vi "Process.vi"(8 "error in":errorcluster, 11 "SMO.A":refnum<class "SMO.Configurable.lvclass">) -> (0 "error out":errorcluster, 3 "SMO.A out":refnum<class "SMO.Configurable.lvclass">)   [LabVIEW 2013, in "SMO.Configurable.lvclass"]
doc: "---------------------------------------------------------------\nJKI State Machine Objects™\nhttp://jki.net/state-machine-objects/\nCopyright (C) 2005-2015, JKI <info@jki.net>\nALL RIGHTS RESERVED"
uses:
  SMO.Configurable.lvclass
  src/SMO/Typedefs/Parent Call--Enum.ctl
  src/SMO/SMO.lvclass
panel:
  # "For instructions on how to use the JKI State Machine Objects, examples and video tutorials, visit:\nhttp://jki.net/state-machine-objects/\n\nJKI State Machine Objects™\nhttp://jki.net/state-machine-objects/\nCopyright (C) 2005-2015, JKI <info@jki.net>\nALL RIGHTS RESERVED"
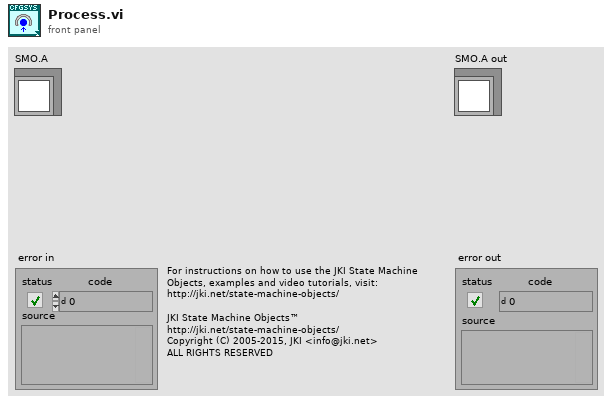
[diagram p1: front panel]
types:
  T1 = typedef "SMO.lvclass/Parent Call--Enum.ctl" = enum16{"Allows parent to run", "Does not request parent to run"}
  T2 = enum32{"invalid app kind", "Development System", "Run Time System", "Student Edition", "Embedded LabVIEW", "Evaluation", "Custom"}
  T3 = enum32{"Invalid", "Standard", "Closed", "Hidden", "Minimized", "Maximized"}
  T4 = cluster{"Core":cluster{"Current VI Reference":refnum<vi>, "Close Panel on Exit?":bool, "error":errorcluster}, "Self Ref":refnum<class "SMO.Configurable.lvclass">, "timeout":i32, "start time":timestamp}
  T5 = cluster{"Current VI Reference":refnum<vi>, "Close Panel on Exit?":bool, "error":errorcluster}
  T6 = typedef "SMO.Configurable.lvclass/Config--cluster.ctl" = cluster{"timeout":i32, "run":bool}
  T7 = typedef "SMO.lvclass/Protected Events.ctl" = cluster{"StopProcesses":refnum<user-event>, "AbortProcesses":refnum<user-event>, "Config Changed":refnum<user-event>, "Dependency":refnum<user-event>}
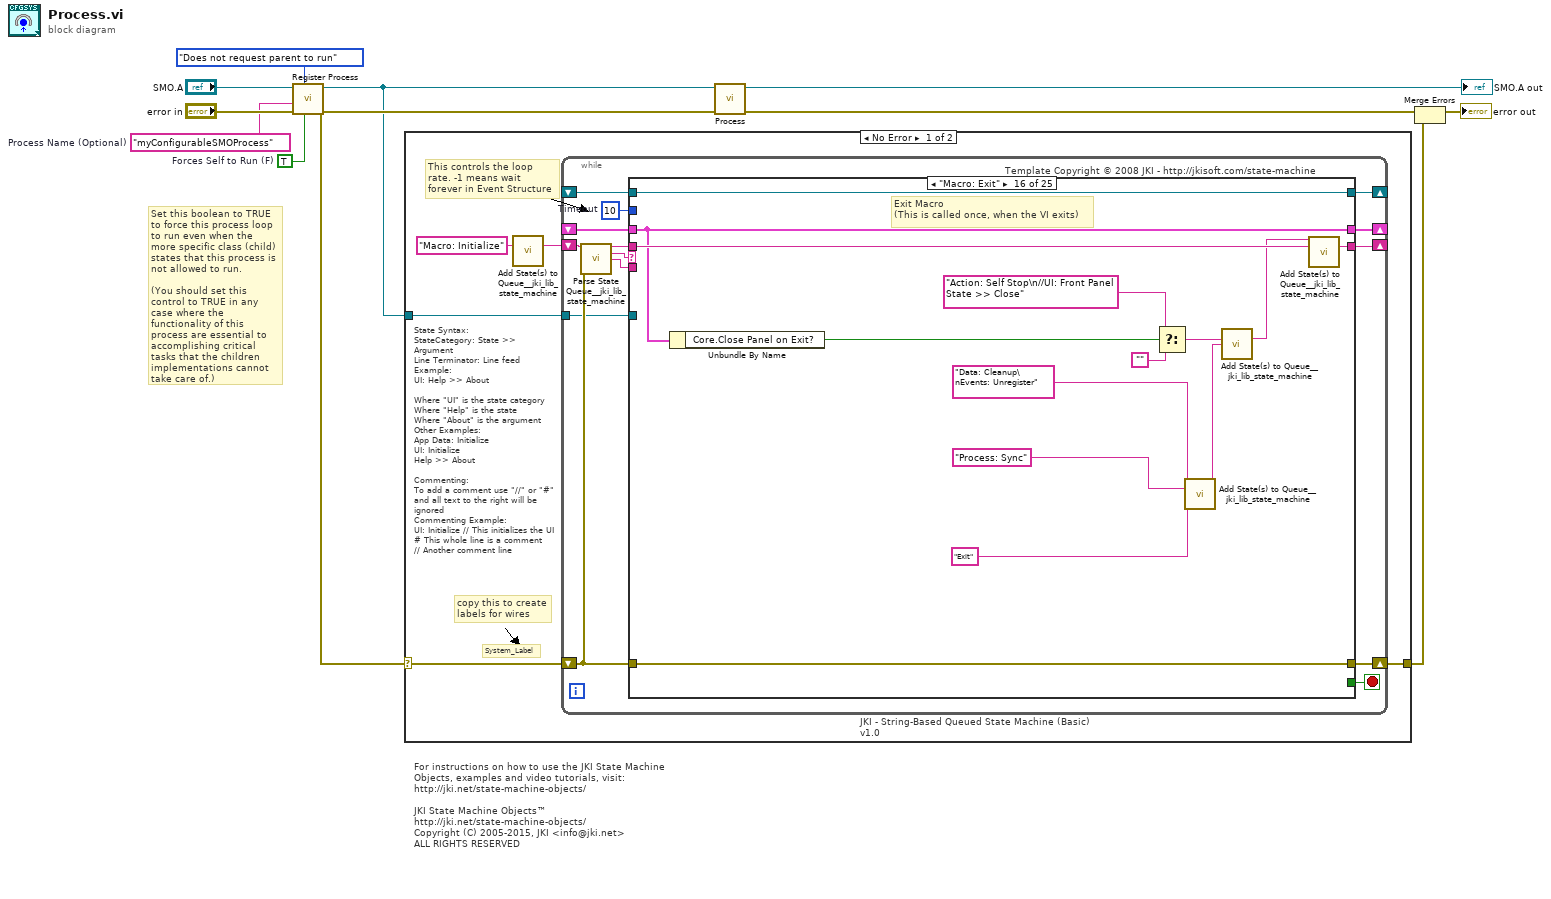
[diagram p0: block diagram]
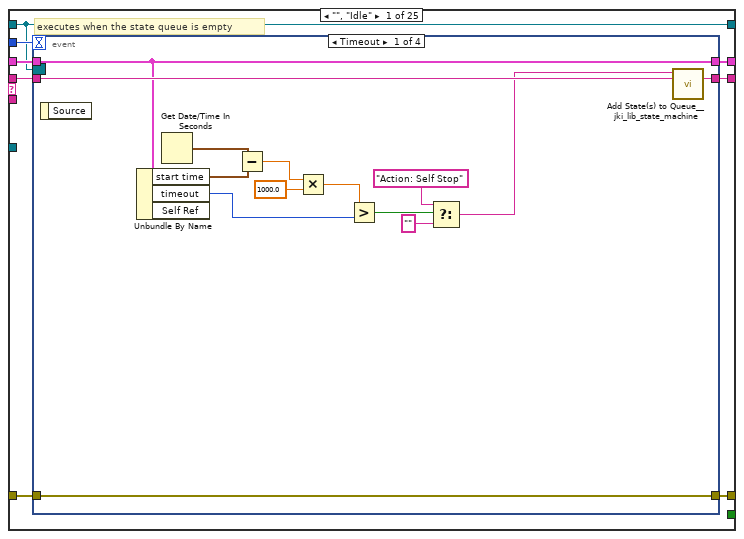
[diagram p2: hidden frame]
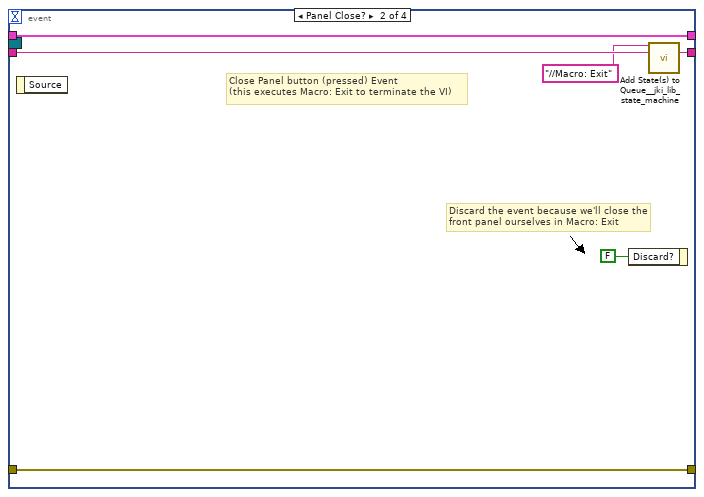
[diagram p3: hidden frame]
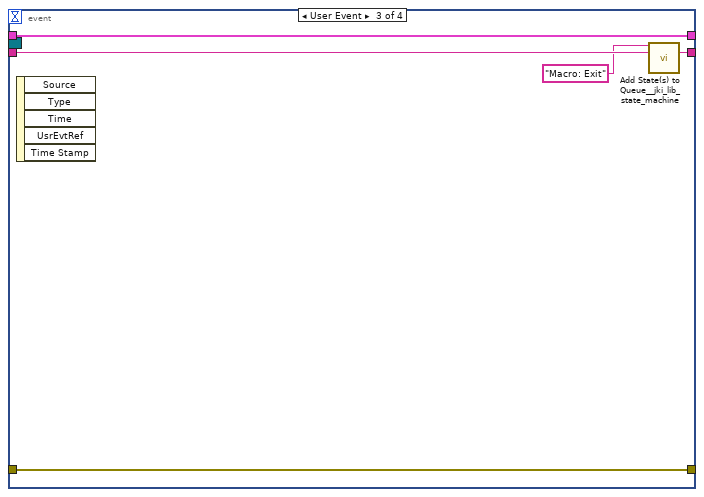
[diagram p4: hidden frame]
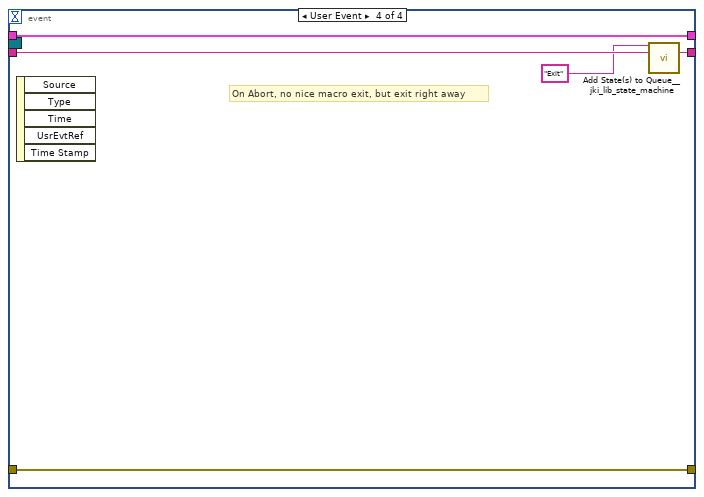
[diagram p5: hidden frame]
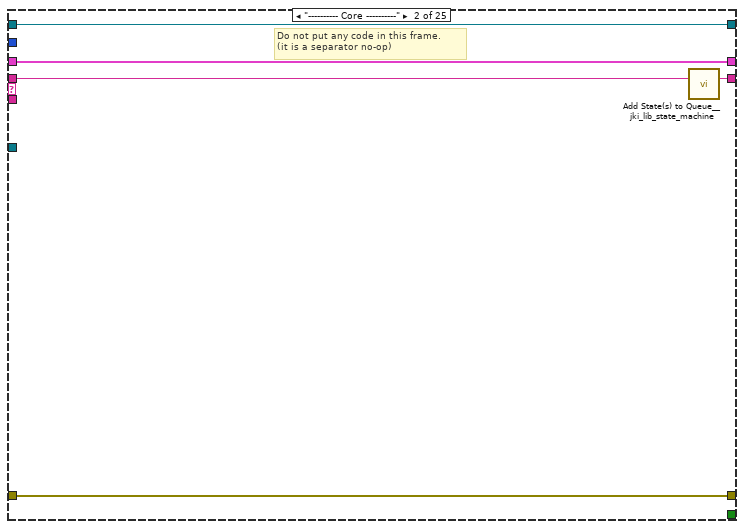
[diagram p6: hidden frame]
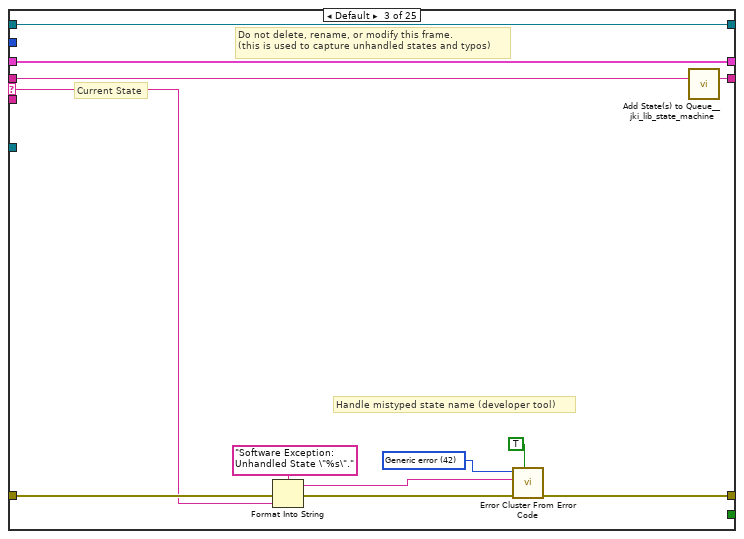
[diagram p7: hidden frame]
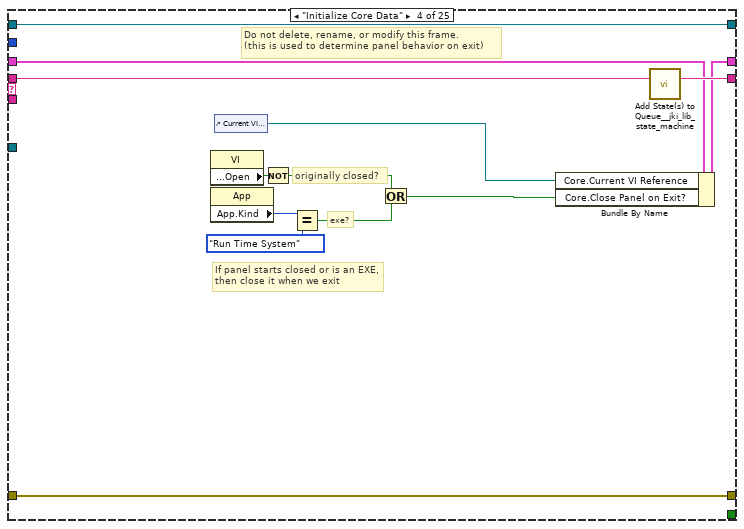
[diagram p8: hidden frame]
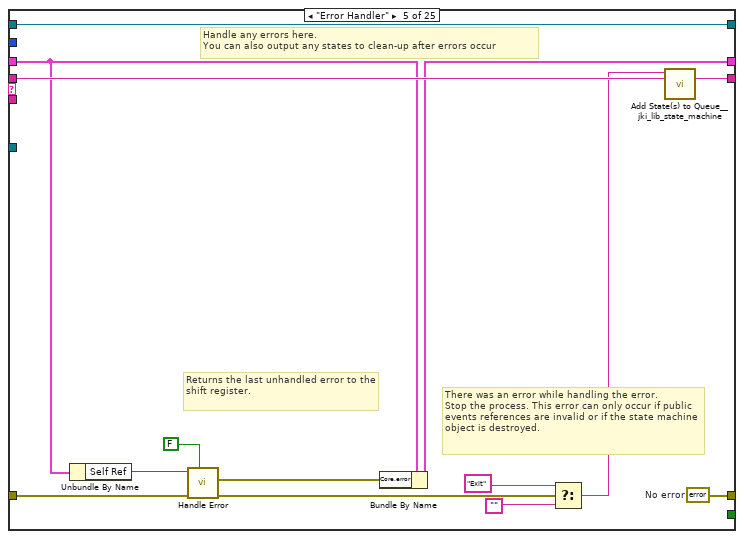
[diagram p9: hidden frame]
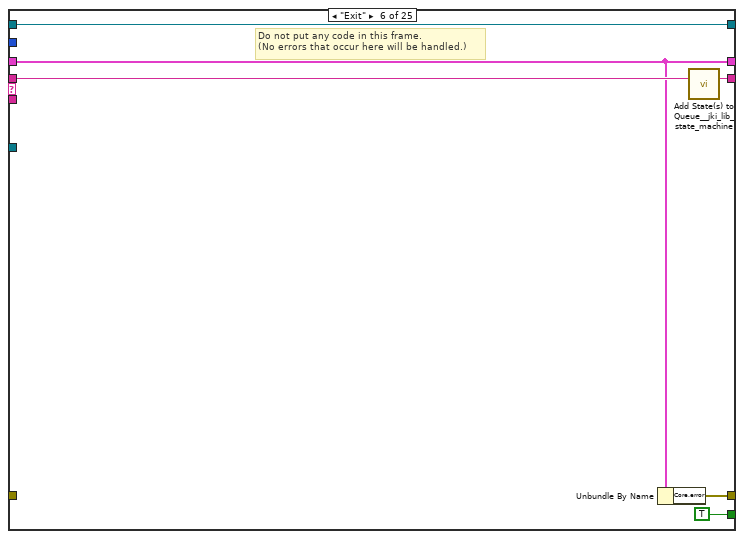
[diagram p10: hidden frame]
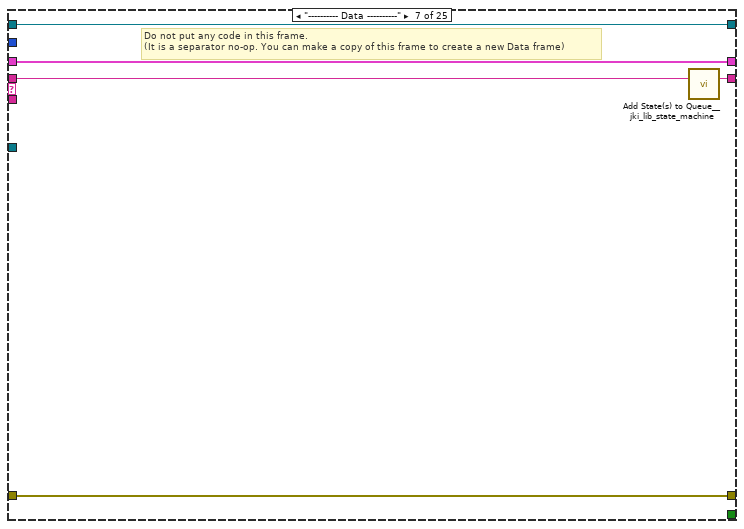
[diagram p11: hidden frame]
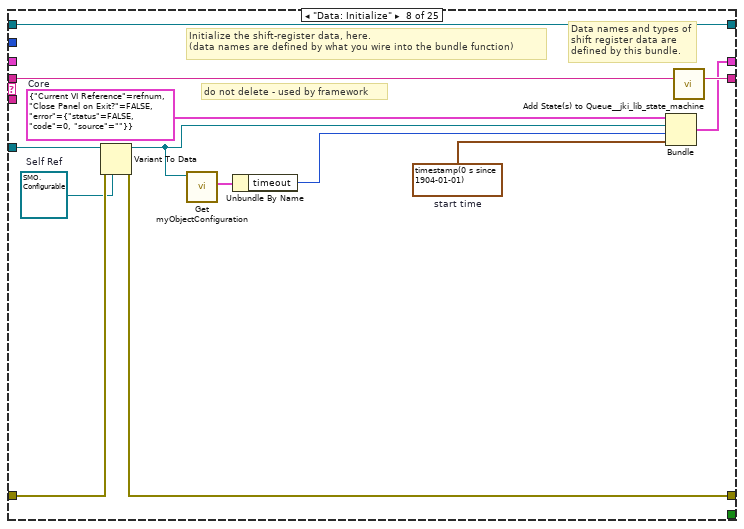
[diagram p12: hidden frame]
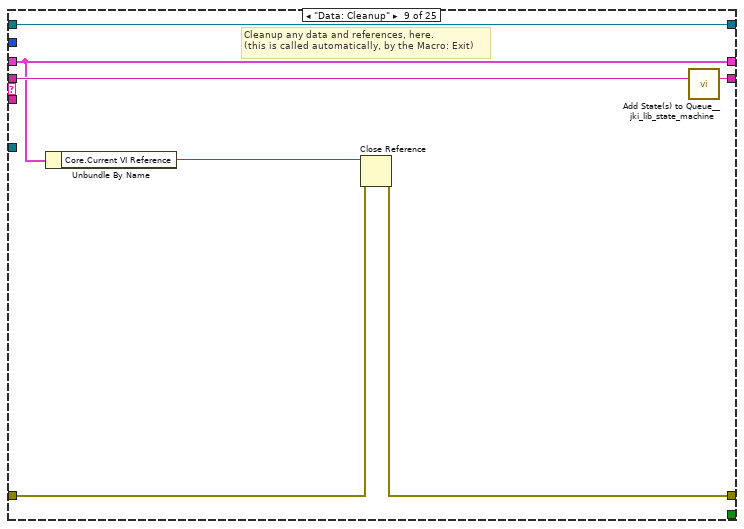
[diagram p13: hidden frame]
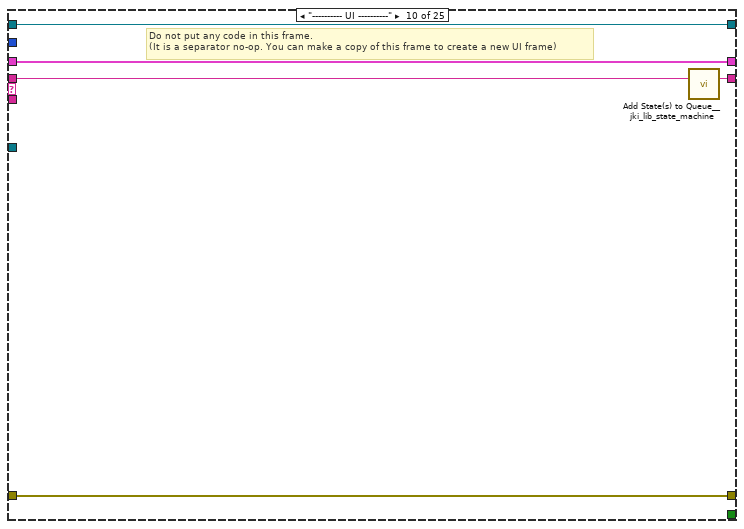
[diagram p14: hidden frame]
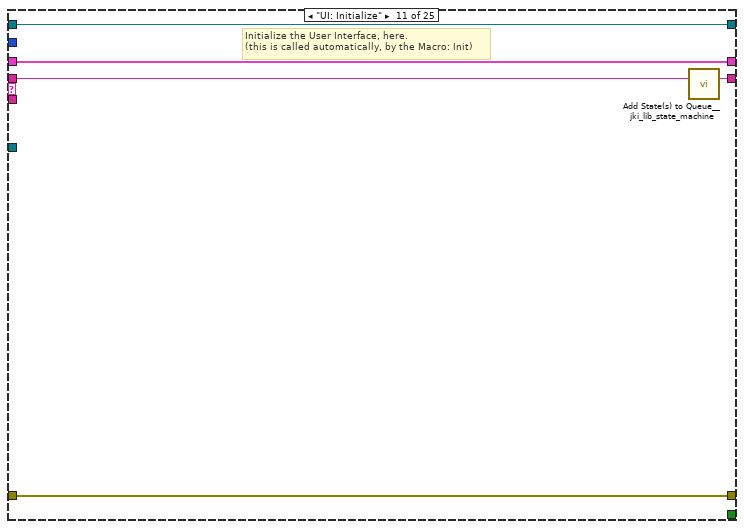
[diagram p15: hidden frame]
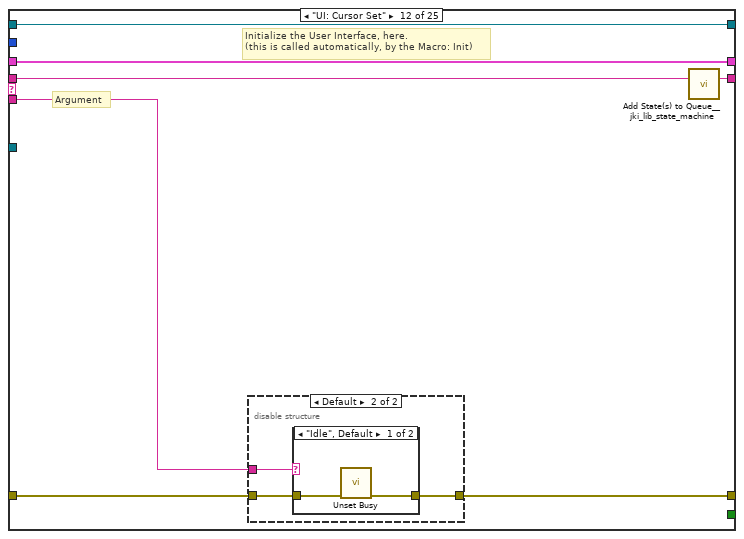
[diagram p16: hidden frame]
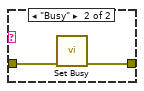
[diagram p18: hidden frame]
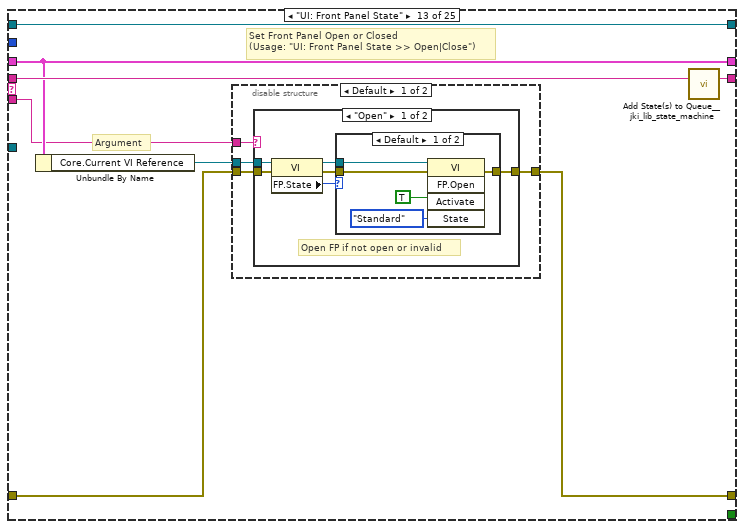
[diagram p19: hidden frame]
diagram:
  w1 = TRUE  # Forces Self to Run (F)
  w2 = "myConfigurableSMOProcess"  # Process Name (Optional)
  # "Set this boolean to TRUE to force this process loop to run even when the more specific class (child) states that this process is not allowed to run.\n\n(You should set this control to TRUE in any case where the functionality of this process are essential to accomplishing critical tasks that the children implementations cannot take care of.)"
  # "For instructions on how to use the JKI State Machine Objects, examples and video tutorials, visit:\nhttp://jki.net/state-machine-objects/\n\nJKI State Machine Objects™\nhttp://jki.net/state-machine-objects/\nCopyright (C) 2005-2015, JKI <info@jki.net>\nALL RIGHTS RESERVED"
  n1 = call "Register Process.vi"("Forces Self to Run (F)"=w1, "Parent Call"=Parent_Call--Enum."Does not request parent to run", "error in (no error)"="error in", "Process Name (optional)"=w2, "SMO"="SMO.A") -> ("error out"=w8:errorcluster, "SMO out"=w7:refnum<class "SMO.Configurable.lvclass">)  [unwired: 5 in]
  n2 = case shown="No Error" w8 {
    selector: w8 -> [w13 w301]
    tunnel: w7 -> [w14 _]
    tunnel: [w12 w301] -> w4
    frame No Error {
      # "State Syntax:\nStateCategory: State >> Argument\nLine Terminator: Line feed\nExample:\nUI: Help >> About\n\nWhere \"UI\" is the state category\nWhere \"Help\" is the state\nWhere \"About\" is the argument\nOther Examples:\nApp Data: Initialize\nUI: Initialize\nHelp >> About\n\nCommenting:\nTo add a comment use \"//\" or \"#\" and all text to the right will be ignored\nCommenting Example:\nUI: Initialize // This initializes the UI\n# This whole line is a comment\n// Another comment line"
      # "copy this to create labels for wires"
      # "This controls the loop rate. -1 means wait forever in Event Structure"
      # "System_Label"
      n3 = call <vilib>:"Add State(s) to Queue__jki_lib_state_machine.vi"("State(s) in (\"\")"="Macro: Initialize") -> ("States Out"=w16:string)  [unwired: 14 in]
      n4 = while "JKI - String-Based Queued State Machine (Basic) v1.0" {
        shift-right: [w23] -> _
        shift-left: _ -> [w22]
        shift-right: [w26] -> w12
        shift-left: w13 -> [w20]
        shift-right: [w25] -> _
        shift-left: w16 -> [w27]
        tunnel: w14 -> [w19]
        shift-right: [w18] -> _
        shift-left: _ -> [w17]
        stop <- w24 stop-if-true
        w21 = 10  # Timeout
        # "Template Copyright © 2008 JKI - http://jkisoft.com/state-machine"
        n5 = call <vilib>:"Parse State Queue__jki_lib_state_machine.vi"("State Queue"=w27, "Error In (no error)"=w20) -> ("Remaining States"=w29:string, "Current State"=w30:string, "Arguments"=w28:string)  [unwired: 11 in]
        n6 = case shown="\"Macro: Exit\"" w30 {
          selector: w30 -> [_ _ w75 _ _ _ _ _ _ _ _ _ _ _ _ _ _ _ _ _ _ _ _ _ _]
          tunnel: w29 -> [w38 w73 w79 w98 w112 w118 w123 w136 w143 w148 w153 w160 w176 w208 w217 w231 w236 w247 w252 w262 w268 w273 w280 w292 w300]
          tunnel: w28 -> [_ _ _ _ _ _ _ _ _ _ _ w154 w169 _ _ _ _ _ _ _ _ _ _ _ _]
          tunnel: w22 -> [w36 w70 w77 w89 w103 w114 w120 _ w138 w145 w151 w158 w174 w205 w213 w222 w233 w244 w249 w260 w266 w271 w275 w289 w297]
          tunnel: [w35 w71 w81 w95 w100 w113 w121 w132 w139 w146 w150 w155 w170 w206 w215 w229 w234 w238 w250 w254 w264 w269 w277 w281 w294] -> w26
          tunnel: w20 -> [w34 w71 w80 w95 w104 _ w121 w133 w140 w146 w150 w156 w171 w206 w215 w229 w234 w239 w250 w255 w264 w269 w277 w282 w295]
          tunnel: [w37 w72 w78 w97 w111 w117 w122 w135 w142 w147 w152 w159 w175 w207 w216 w230 w235 w246 w251 w261 w267 w272 w279 w291 w299] -> w25
          tunnel: [_ _ _ _ _ TRUE _ _ _ _ _ _ _ _ _ _ _ _ _ _ _ _ _ _ _] -> w24
          tunnel: [w33 w70 w77 w96 w102 w114 w120 w134 w138 w145 w151 w158 w174 w205 w213 w222 w233 w244 w249 w260 w266 w271 w274 w289 w297] -> w23
          tunnel: w21 -> [w32 _ _ _ _ _ _ _ _ _ _ _ _ _ _ _ _ _ _ _ _ _ _ _ _]
          tunnel: w19 -> [_ _ _ _ _ _ _ w130 _ _ _ _ _ _ _ _ _ _ _ _ _ _ _ _ _]
          tunnel: [w31 w69 w74 w86 w110 w115 w119 w129 w137 w144 w149 w157 w173 w204 w214 w223 w232 w245 w248 w258 w265 w270 w278 w290 w298] -> w18
          tunnel: w17 -> [w31 w69 w74 w86 w110 w115 w119 w129 w137 w144 w149 w157 w173 w204 w214 w223 w232 w245 w248 _ w265 w270 w278 w290 w298]
          frame "", "Idle" {
            # "executes when the state queue is empty"
            n7 = event shown="[0] Timeout" {
              selector: w31 -> [_ _ _ _]
              dyn-events: _ -> [_ _ _ _]
              timeout: w32 -> [_ _ _ _]
              tunnel: w38 -> [w52 w58 w63 w68]
              tunnel: [w51 w57 w62 w67] -> w37
              tunnel: w36 -> [w49 w55 w60 w65]
              tunnel: [w50 w56 w61 w66] -> w35
              tunnel: w34 -> [w50 w56 w61 w66]
              tunnel: [w49 w55 w60 w65] -> w33
              event Timeout {
                n8 = event-data() -> ()  [unwired: 1 in, 1 out]
                n9 = Unbundle By Name(w49) -> ("start time"=w47:timestamp, "timeout"=w43:i32)  [unwired: 1 out]
                n10 = Get Date/Time In Seconds() -> (seconds since 1Jan1904=w48:timestamp)
                n11 = Subtract(x=w48, y=w47) -> (x-y=w45:dbl)
                n12 = Multiply(x=w45, y=1000.0) -> (x*y=w44:dbl)
                n13 = Greater?(x=w44, y=w43) -> (0:w42:bool)
                n14 = Select(t="Action: Self Stop", s=w42, f="") -> (s? t:f=w39:string)
                n15 = call <vilib>:"Add State(s) to Queue__jki_lib_state_machine.vi"("State(s) in Front (\"\")"=w39, "State(s) in (\"\")"=w52) -> ("States Out"=w51:string)  [unwired: 13 in]
              }
              event Panel Close? {
                # "Discard the event because we'll close the front panel ourselves in Macro: Exit"
                # "Close Panel button (pressed) Event\n(this executes Macro: Exit to terminate the VI)"
                n16 = event-data() -> ()  [unwired: 1 in, 1 out]
                n17 = event-data("Discard?"=FALSE) -> ()  [unwired: 1 in, 1 out]
                n18 = call <vilib>:"Add State(s) to Queue__jki_lib_state_machine.vi"("State(s) in Front (\"\")"="//Macro: Exit", "State(s) in (\"\")"=w58) -> ("States Out"=w57:string)  [unwired: 13 in]
              }
              event User Event {
                n19 = event-data() -> ()  [unwired: 1 in, 5 out]
                n20 = call <vilib>:"Add State(s) to Queue__jki_lib_state_machine.vi"("State(s) in Front (\"\")"="Macro: Exit", "State(s) in (\"\")"=w63) -> ("States Out"=w62:string)  [unwired: 13 in]
              }
              event User Event {
                # "On Abort, no nice macro exit, but exit right away"
                n21 = event-data() -> ()  [unwired: 1 in, 5 out]
                n22 = call <vilib>:"Add State(s) to Queue__jki_lib_state_machine.vi"("State(s) in Front (\"\")"="Exit", "State(s) in (\"\")"=w68) -> ("States Out"=w67:string)  [unwired: 13 in]
              }
            }
          }
          frame "---------- Core ----------" {
            # "Do not put any code in this frame.\n(it is a separator no-op)"
            n23 = call <vilib>:"Add State(s) to Queue__jki_lib_state_machine.vi"("State(s) in (\"\")"=w73) -> ("States Out"=w72:string)  [unwired: 14 in]
          }
          frame Default {
            w84 = 42 items=["No error", "Argument error", "Memory is full", "Out of zone", "End of file", "File already open", "Generic file I/O error", "File not found", "File permission error", "Disk is full", "Duplicate path", "Too many files open", "System feature not enabled", "Resource file not found", "Cannot add resource", "Resource not found", "Image not found", "Image memory error", "Pen does not exist", "Config type invalid", "Config token not found", "Config parse error", "Config memory error", "Bad external code format", "Bad external code offset", "External code not present", "Null window", "Destroy window error", "Null menu", "Print aborted", "Bad print record", "Print driver error", "Windows error during printing", "Memory error during printing", "Print dialog error", "Generic print error", "Invalid device refnum", "Device not found", "Device parameter error", "Device unit error", "Cannot open device", "Device call aborted", "Generic error", "Cancelled by user", "Object ID too low", "Object ID too high", "Object not in heap", "Unknown heap", "Unknown object (invalid DefProc)", "Unknown object (DefProc not in table)", "Message out of range", "Invalid (null) method", "Unknown message", "Manager call not supported", "Bad address", "Network operation in progress", "Network operation timed out", "Connection is busy", "Network attribute not supported", "Network error", "Address in use", "System out of memory", "Connection aborted", "Connection refused", "Not connected", "Already connected", "Connection closed", "Initialization error (interapplication manager)", "Bad occurrence", "Wait on unbound occurrence handler", "Occurrence queue overflow", "Datalog type conflict", "Unused", "Unrecognized type (interapplication manager)", "Memory corrupt", "Failed to make temporary DLL", "Old CIN version", "Drag socket not found", "Failed to load drop-object", "Failed to register OLE object", "Failed to release OLE object", "Format specifier type mismatch", "Unknown format specifier", "Too few format specifiers", "Too many format specifiers", "Scan failed", "Newer CIN version", "Error converting to variant", "Runtime menu error", "Password tampered", "Variant attribute not found", "Incompatible variant data type", "Event data is not available", "Event Store is not present", "Occurrence is not found", "Event Queue is not created", "Event info is not available", "Refnum passed is NULL", "Error retrieving Class GUID", "Error retrieving CoClass GUID", "Error retrieving TypeLib GUID.", "Bad built application magic bytes.", "Specific driver is different from the specific driver associated with the Logical Name.", "There is no session opened to the class driver.", "Max Error", "MAX - Error with config objects", "MAX - Error loading configuration", "MAX - Group not supported"]
            # "Current State"
            # "Do not delete, rename, or modify this frame.\n(this is used to capture unhandled states and typos)"
            # "Handle mistyped state name (developer tool)"
            n24 = Format Into String(format string="Software Exception: Unhandled State \"%s\"." ("message"), error in=w80, w75) -> (resulting string=w83:string, error out=w82:errorcluster)  [unwired: 1 in]
            n25 = call <vilib>:"Error Cluster From Error Code.vi"("show call chain? (False)"=TRUE, "error in (no error)"=w82, "error message (\"\")"=w83, "error code (0)"=w84) -> ("error out"=w81:errorcluster)  [unwired: 5 in]
            n26 = call <vilib>:"Add State(s) to Queue__jki_lib_state_machine.vi"("State(s) in (\"\")"=w79) -> ("States Out"=w78:string)  [unwired: 14 in]
          }
          frame "Initialize Core Data" {
            # "Do not delete, rename, or modify this frame.\n(this is used to determine panel behavior on exit)"
            # "originally closed?"
            # "exe?"
            # "If panel starts closed or is an EXE, then close it when we exit"
            n27 = property class="VI"() -> ("Front Panel.Open"=w94:bool)  [unwired: 2 in, 2 out]
            n28 = property class="App"() -> ("App.Kind"=w93:T2)  [unwired: 2 in, 2 out]
            n29 = control-ref of="Current VI Reference"() -> (w87:refnum<vi>)
            n30 = Not(x=w94) -> (.not. x?=w91:bool)
            n31 = Equal?(x=w93, y=T2."Run Time System" ("Application:Kind")) -> (x = y?=w90:bool)
            n32 = Or(x=w91, y=w90) -> (x .or. y?=w88:bool)
            n33 = Bundle By Name(cluster=w89, "Core.Current VI Reference"=w87, "Core.Close Panel on Exit?"=w88) -> (w96:T4)
            n34 = call <vilib>:"Add State(s) to Queue__jki_lib_state_machine.vi"("State(s) in (\"\")"=w98) -> ("States Out"=w97:string)  [unwired: 14 in]
          }
          frame "Error Handler" {
            w100 = errorcluster {"status"=FALSE, "code"=0, "source"=""}  # No error
            # "Returns the last unhandled error to the shift register."
            # "There was an error while handling the error.\nStop the process. This error can only occur if public events references are invalid or if the state machine object is destroyed."
            # "Handle any errors here.\nYou can also output any states to clean-up after errors occur"
            n35 = Unbundle By Name(w103) -> ("Self Ref"=w105:refnum<class "SMO.Configurable.lvclass">)
            n36 = call-dynamic "Handle Error.vi"("Stop on Unhandled Error (T)"=FALSE, "error in"=w104, "SMO"=w105) -> ("handling error"=w107:errorcluster, "Unhandled error"=w106:errorcluster)  [unwired: 6 in, 1 out]
            n37 = Bundle By Name(cluster=w103, "Core.error"=w106) -> (w102:T4)
            n38 = Select(t="Exit", s=w107, f="") -> (s? t:f=w101:string)
            n39 = call <vilib>:"Add State(s) to Queue__jki_lib_state_machine.vi"("State(s) in Front (\"\")"=w101, "State(s) in (\"\")"=w112) -> ("States Out"=w111:string)  [unwired: 13 in]
          }
          frame "Exit" {
            # "Do not put any code in this frame.\n(No errors that occur here will be handled.)"
            n40 = Unbundle By Name(w114) -> ("Core.error"=w113:errorcluster)
            n41 = call <vilib>:"Add State(s) to Queue__jki_lib_state_machine.vi"("State(s) in (\"\")"=w118) -> ("States Out"=w117:string)  [unwired: 14 in]
          }
          frame "---------- Data ----------" {
            # "Do not put any code in this frame.\n(It is a separator no-op. You can make a copy of this frame to create a new Data frame)"
            n42 = call <vilib>:"Add State(s) to Queue__jki_lib_state_machine.vi"("State(s) in (\"\")"=w123) -> ("States Out"=w122:string)  [unwired: 14 in]
          }
          frame "Data: Initialize" {
            w124 = timestamp(0 s since 1904-01-01)  # start time
            w128 = T5 {"Current VI Reference"=refnum, "Close Panel on Exit?"=FALSE, "error"={"status"=FALSE, "code"=0, "source"=""}}  # Core
            w131 = refnum<class "SMO.Configurable.lvclass"> refnum  # Self Ref
            # "do not delete - used by framework"
            # "Data names and types of shift register data are defined by this bundle."
            # "Initialize the shift-register data, here.\n(data names are defined by what you wire into the bundle function)"
            n43 = Variant To Data(error in=w133, type=w131, Variant=w130) -> (data=w127:refnum<class "SMO.Configurable.lvclass">, error out=w132:errorcluster)
            n44 = call "Get myObjectConfiguration.vi"("SMO.Configurable in"=w127) -> ("Config"=w126:T6)  [unwired: 8 in, 2 out]
            n45 = Unbundle By Name(w126) -> ("timeout"=w125:i32)
            n46 = Bundle("Core"=w128, "Self Ref"=w127, "timeout"=w125, "start time"=w124) -> (w134:T4)  [unwired: 1 in]
            n47 = call <vilib>:"Add State(s) to Queue__jki_lib_state_machine.vi"("State(s) in (\"\")"=w136) -> ("States Out"=w135:string)  [unwired: 14 in]
          }
          frame "Data: Cleanup" {
            # "Cleanup any data and references, here.\n(this is called automatically, by the Macro: Exit)"
            n48 = Unbundle By Name(w138) -> ("Core.Current VI Reference"=w141:refnum<vi>)
            n49 = Close Reference(reference=w141, error in (no error)=w140) -> (error out=w139:errorcluster)
            n50 = call <vilib>:"Add State(s) to Queue__jki_lib_state_machine.vi"("State(s) in (\"\")"=w143) -> ("States Out"=w142:string)  [unwired: 14 in]
          }
          frame "---------- UI ----------" {
            # "Do not put any code in this frame.\n(It is a separator no-op. You can make a copy of this frame to create a new UI frame)"
            n51 = call <vilib>:"Add State(s) to Queue__jki_lib_state_machine.vi"("State(s) in (\"\")"=w148) -> ("States Out"=w147:string)  [unwired: 14 in]
          }
          frame "UI: Initialize" {
            # "Initialize the User Interface, here.\n(this is called automatically, by the Macro: Init)"
            n52 = call <vilib>:"Add State(s) to Queue__jki_lib_state_machine.vi"("State(s) in (\"\")"=w153) -> ("States Out"=w152:string)  [unwired: 14 in]
          }
          frame "UI: Cursor Set" {
            # "Argument"
            # "Initialize the User Interface, here.\n(this is called automatically, by the Macro: Init)"
            n53 = disable-structure shown="Default" {
              disable-tunnel: w156 -> [w161 w164]
              disable-tunnel: [w161 w163] -> w155
              disable-tunnel: w154 -> [_ w162]
              frame condition #0 {
              }
              frame condition #1 (active) {
                n54 = case shown="\"Idle\", Default" w162 {
                  tunnel: w164 -> [w166 w168]
                  tunnel: [w165 w167] -> w163
                  frame "Idle", Default {
                    n55 = call <vilib>:"Unset Busy.vi"("error in (no error)"=w166) -> ("error out"=w165:errorcluster)  [unwired: 10 in]
                  }
                  frame "Busy" {
                    n56 = call <vilib>:"Set Busy.vi"("error in (no error)"=w168) -> ("error out"=w167:errorcluster)  [unwired: 9 in, 1 out]
                  }
                }
              }
            }
            n57 = call <vilib>:"Add State(s) to Queue__jki_lib_state_machine.vi"("State(s) in (\"\")"=w160) -> ("States Out"=w159:string)  [unwired: 14 in]
          }
          frame "UI: Front Panel State" {
            # "Argument"
            # "Set Front Panel Open or Closed\n(Usage: \"UI: Front Panel State >> Open|Close\")"
            n58 = Unbundle By Name(w174) -> ("Core.Current VI Reference"=w172:refnum<vi>)
            n59 = disable-structure shown="Default" {
              disable-tunnel: w171 -> [w180 w203]
              disable-tunnel: [w179 w203] -> w170
              disable-tunnel: w172 -> [w178 _]
              disable-tunnel: w169 -> [w177 _]
              frame condition #0 (active) {
                n60 = case shown="\"Open\"" w177 {
                  tunnel: w180 -> [w184 w197]
                  tunnel: [w186 w198] -> w179
                  tunnel: w178 -> [w185 w195]
                  frame "Open" {
                    # "Open FP if not open or invalid"
                    n61 = property class="VI"(reference=w185, error in=w184) -> (reference out=w182:refnum<vi>, error out=w183:errorcluster, "FP.State"=w181:T3)
                    n62 = case shown="Default" w181 {
                      tunnel: [w189 w192] -> w186
                      tunnel: w183 -> [w188 w192]
                      tunnel: w182 -> [w187 _]
                      frame Default {
                        n63 = invoke class="VI" method="FP.Open"(reference=w187, error in=w188, "Activate"=TRUE, "State"=T3."Standard") -> (error out=w189:errorcluster)  [unwired: 1 in, 4 out]
                      }
                      frame "Invalid", "Standard" {
                      }
                    }
                  }
                  frame "Close", Default {
                    # "Close FP is not Closed or Invalid"
                    n64 = property class="VI"(reference=w195, error in=w197) -> (reference out=w194:refnum<vi>, error out=w196:errorcluster, "FP.State"=w193:T3)
                    n65 = case shown="Default" w193 {
                      tunnel: [w199 w202] -> w198
                      tunnel: w196 -> [w199 w201]
                      tunnel: w194 -> [_ w200]
                      frame "Invalid", "Closed" {
                      }
                      frame Default {
                        n66 = invoke class="VI" method="FP.Close"(reference=w200, error in=w201) -> (error out=w202:errorcluster)  [unwired: 1 in, 2 out]
                      }
                    }
                  }
                }
              }
              frame condition #1 {
              }
            }
            n67 = call <vilib>:"Add State(s) to Queue__jki_lib_state_machine.vi"("State(s) in (\"\")"=w176) -> ("States Out"=w175:string)  [unwired: 14 in]
          }
          frame "---------- Macro ----------" {
            # "Do not put any code in this frame.\n(It is a separator no-op. You can make a copy of this frame to create a new Macro frame)"
            n68 = call <vilib>:"Add State(s) to Queue__jki_lib_state_machine.vi"("State(s) in (\"\")"=w208) -> ("States Out"=w207:string)  [unwired: 14 in]
          }
          frame "Macro: Initialize" {
            w211 = "UI: Initialize\n//UI: Front Panel State >> Open\nAction: Initialize Timer\nAction: Check Dependency Status"  # UI: Initialize //UI: Front Panel State >> Open Action: Initialize Timer Action: Check Dependency Status
            # "Initialization Macro\n(This is called once, when the VI starts)"
            n69 = call <vilib>:"Add State(s) to Queue__jki_lib_state_machine.vi"("State(s) in Front (\"\")"="Data: Initialize\nInitialize Core Data\nEvents: Register", "State(s) in (\"\")"="Process: Sync", "State(s) at Back (\"\")"=w211) -> ("States Out"=w210:string)  [unwired: 12 in]
            n70 = call <vilib>:"Add State(s) to Queue__jki_lib_state_machine.vi"("State(s) in Front (\"\")"=w210, "State(s) in (\"\")"=w217) -> ("States Out"=w216:string)  [unwired: 13 in]
          }
          frame "Macro: Exit" {
            # "Exit Macro\n(This is called once, when the VI exits)"
            n71 = Unbundle By Name(w222) -> ("Core.Close Panel on Exit?"=w228:bool)
            n72 = Select(t="Action: Self Stop\n//UI: Front Panel State >> Close", s=w228, f="") -> (s? t:f=w225:string)
            n73 = call <vilib>:"Add State(s) to Queue__jki_lib_state_machine.vi"("State(s) in Front (\"\")"="Data: Cleanup\nEvents: Unregister", "State(s) in (\"\")"="Process: Sync", "State(s) at Back (\"\")"="Exit") -> ("States Out"=w219:string)  [unwired: 12 in]
            n74 = call <vilib>:"Add State(s) to Queue__jki_lib_state_machine.vi"("State(s) in (\"\")"=w225, "State(s) at Back (\"\")"=w219) -> ("States Out"=w224:string)  [unwired: 13 in]
            n75 = call <vilib>:"Add State(s) to Queue__jki_lib_state_machine.vi"("State(s) in Front (\"\")"=w224, "State(s) in (\"\")"=w231) -> ("States Out"=w230:string)  [unwired: 13 in]
          }
          frame "---------- Process ----------" {
            # "Template Separator\n(You can make a copy of, or modify, this frame)"
            n76 = call <vilib>:"Add State(s) to Queue__jki_lib_state_machine.vi"("State(s) in (\"\")"=w236) -> ("States Out"=w235:string)  [unwired: 14 in]
          }
          frame "Process: Sync" {
            # "Template Separator\n(You can make a copy of, or modify, this frame)"
            n77 = Unbundle By Name(w244) -> ("Self Ref"=w240:refnum<class "SMO.Configurable.lvclass">)
            n78 = call "WaitOnProcessSync.vi"("error in (no error)"=w239, "SMO"=w240) -> ("error out"=w238:errorcluster, "Don't run?"=w243:bool)  [unwired: 7 in, 1 out]
            n79 = Select(t="Data: Cleanup\nEvents: Unregister\nExit", s=w243, f="") -> (s? t:f=w237:string)
            n80 = call <vilib>:"Add State(s) to Queue__jki_lib_state_machine.vi"("State(s) in Front (\"\")"=w237, "State(s) in (\"\")"=w247) -> ("States Out"=w246:string)  [unwired: 13 in]
          }
          frame "---------- Events ----------" {
            # "Template Separator\n(You can make a copy of, or modify, this frame)"
            n81 = call <vilib>:"Add State(s) to Queue__jki_lib_state_machine.vi"("State(s) in (\"\")"=w252) -> ("States Out"=w251:string)  [unwired: 14 in]
          }
          frame "Events: Register" {
            # "Your code here.\n(You can make a copy of, or modify, this frame)"
            n82 = Unbundle By Name(w260) -> ("Self Ref"=w253:refnum<class "SMO.Configurable.lvclass">)
            n83 = call "GetProtectedEvents.vi"("SMO"=w253) -> ("error out"=w256:errorcluster, "SMO Protected Events"=w259:T7)  [unwired: 8 in, 1 out]
            n84 = register-events(w259) -> (reference out=w258:refnum<event-registration>, error out=w257:errorcluster)  [unwired: 2 in]
            n85 = Merge Errors(w255, w257, w256) -> (w254:errorcluster)
            n86 = call <vilib>:"Add State(s) to Queue__jki_lib_state_machine.vi"("State(s) in (\"\")"=w262) -> ("States Out"=w261:string)  [unwired: 14 in]
          }
          frame "Events: Unregister" {
            # "Your code here.\n(You can make a copy of, or modify, this frame)"
            n87 = Unregister For Events(event registration refnum=w265, error in=w264) -> (error out=w263:errorcluster)
            n88 = call <vilib>:"Clear Errors.vi"("error in (no error)"=w263) -> ()  [unwired: 6 in, 1 out]
            n89 = call <vilib>:"Add State(s) to Queue__jki_lib_state_machine.vi"("State(s) in (\"\")"=w268) -> ("States Out"=w267:string)  [unwired: 14 in]
          }
          frame "---------- Action ----------" {
            n90 = call <vilib>:"Add State(s) to Queue__jki_lib_state_machine.vi"("State(s) in (\"\")"=w273) -> ("States Out"=w272:string)  [unwired: 14 in]
          }
          frame "Action: Initialize Timer" {
            n91 = Get Date/Time In Seconds() -> (seconds since 1Jan1904=w276:timestamp)
            n92 = Bundle By Name(cluster=w275, "start time"=w276) -> (w274:T4)
            n93 = call <vilib>:"Add State(s) to Queue__jki_lib_state_machine.vi"("State(s) in (\"\")"=w280) -> ("States Out"=w279:string)  [unwired: 14 in]
          }
          frame "Action: Check Dependency Status" {
            n94 = Unbundle By Name(w289) -> ("Self Ref"=w286:refnum<class "SMO.Configurable.lvclass">)
            n95 = call "ListDependencies.vi"("error in (no error)"=w282, "SMO in"=w286) -> ("error out"=w281:errorcluster, "[Dependencies]"=w284:refnum<class "SMO.lvclass">[])  [unwired: 6 in, 2 out]
            n96 = Empty Array?(array=w284) -> (empty?=w283:bool)
            n97 = Select(t="Macro: Exit", s=w283, f="") -> (s? t:f=w285:string)
            n98 = call <vilib>:"Add State(s) to Queue__jki_lib_state_machine.vi"("State(s) in Front (\"\")"=w285, "State(s) in (\"\")"=w292) -> ("States Out"=w291:string)  [unwired: 13 in]
          }
          frame "Action: Self Stop" {
            n99 = Unbundle By Name(w297) -> ("Self Ref"=w296:refnum<class "SMO.Configurable.lvclass">)
            n100 = call "SelfTerminate.vi"("error in (no error)"=w295, "SMO in"=w296) -> ("error out"=w294:errorcluster)  [unwired: 8 in, 1 out]
            n101 = call <vilib>:"Add State(s) to Queue__jki_lib_state_machine.vi"("State(s) in Front (\"\")"="Macro: Exit", "State(s) in (\"\")"=w300) -> ("States Out"=w299:string)  [unwired: 13 in]
          }
        }
      }
    }
    frame Error {
    }
  }
  n102 = call-parent "Process.vi"("error in"=w8, "SMO"=w7) -> ("error out"=w5:errorcluster, "SMO out"=→"SMO.A out":refnum<class "SMO.Configurable.lvclass">)  [unwired: 8 in]
  n103 = Merge Errors(w5, w4) -> (→"error out":errorcluster)
